vi "OAT Output Trigger Event (time).vi"(0 "signal in":timestamp, 2 "reset? (F)":bool, 5 "time stamp setpoint":timestamp, 11 "error in (no error)":errorcluster) -> (4 "trigger detected?":bool, 15 "error out":errorcluster)   [LabVIEW 2017, in "SoundVib_OAUtility.lvlib"]
doc: "Detects the first level-crossing condition. The <B>upper setpoint</B> and <B>lower setpoint</B> of the threshold and the <B>hysteresis</B> specify the trigger conditions. Wire data to the <B>signal in</B> input to determine the polymorphic instance to use or manually select the instance."
uses:
  <vilib>/addons/Sound and Vibration/Order Analysis/Utility/SoundVib_OAUtility.lvlib
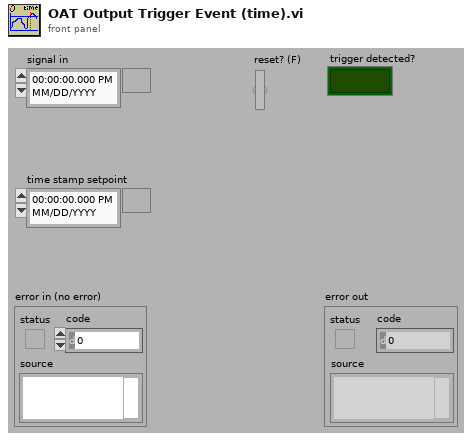
[diagram p1: front panel]
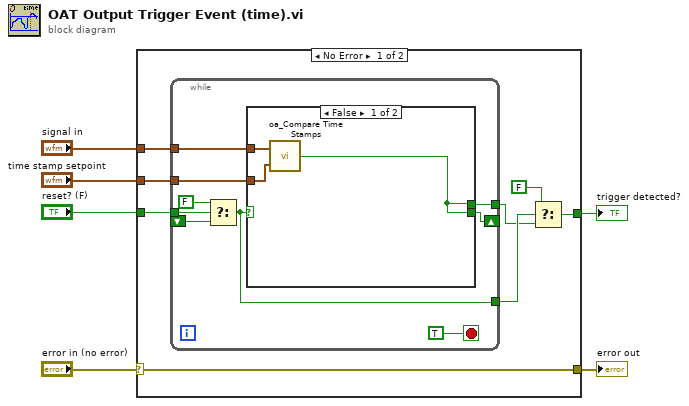
[diagram p0: block diagram]
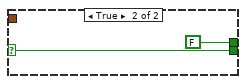
[diagram p2: hidden frame]
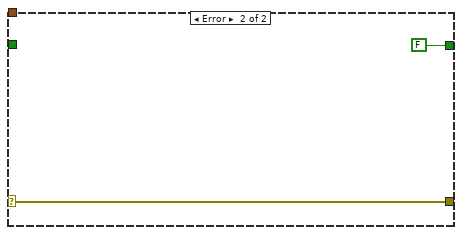
[diagram p3: hidden frame]
diagram:
  n1 = case shown="No Error" "error in (no error)" {
    selector: "error in (no error)" -> [w14 w30]
    tunnel: [w14 w30] -> w5
    tunnel: "signal in" -> [w12 _]
    tunnel: "reset? (F)" -> [w13 _]
    tunnel: "time stamp setpoint" -> [w11 _]
    tunnel: [w9 FALSE ("t")] -> w1
    frame No Error {
      n2 = while {
        shift-right: [w22] -> _
        shift-left: _ -> [w19]
        tunnel: w13 -> [w21]
        tunnel: w12 -> [w18]
        tunnel: w11 -> [w17]
        tunnel: [w16] -> w10
        tunnel: [w15] -> w7
        stop <- TRUE stop-if-true
        n3 = Select(t=FALSE, s=w21, f=w19) -> (s? t:f=w16:bool)
        n4 = case shown="False" w16 {
          selector: w16 -> [_ w28]
          tunnel: [w24 w28] -> w22
          tunnel: w18 -> [w26 _]
          tunnel: w17 -> [w25 _]
          tunnel: [w24 FALSE ("t")] -> w15
          frame False {
            n5 = call <vilib>:"oa_Compare Time Stamps.vi"("time stamp limit"=w25, "time stamp in"=w26) -> ("greater than?"=w24:bool)
          }
          frame True {
          }
        }
      }
      n6 = Select(t=FALSE, s=w10, f=w7) -> (s? t:f=w9:bool)
    }
    frame Error {
    }
  }
  "error out" <- w5
  "trigger detected?" <- w1
